vi "Destroy User Event.vi"(8 "error in (no error)":errorcluster) -> (0 "error out":errorcluster)   [LabVIEW 2017]
uses:
  Reference Action.ctl
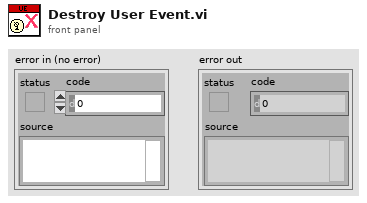
[diagram p1: front panel]
types:
  T1 = typedef "Reference Action.ctl" = enum16{"Set", "Get"}
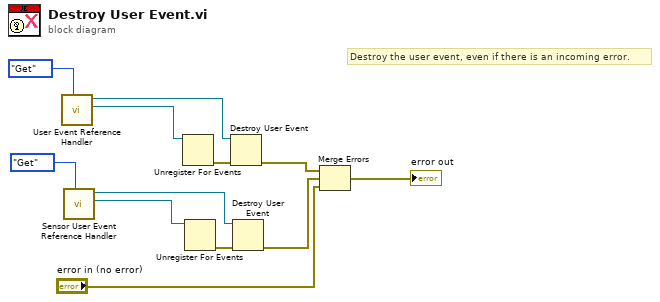
[diagram p0: block diagram]
diagram:
  # "Destroy the user event, even if there is an incoming error."
  n1 = call "User Event Reference Handler.vi"("Reference Action"=Reference_Action."Get") -> ("Event Registration Refnum Out"=w10:refnum<event-registration>, "User Event Refnum Out"=w9:refnum<user-event>)  [unwired: 8 in, 1 out]
  n2 = call "Sensor User Event Reference Handler.vi"("Reference Action"=Reference_Action."Get") -> ("Event Registration Refnum Out"=w3:refnum<event-registration>, "User Event Refnum Out"=w4:refnum<user-event>)  [unwired: 8 in, 1 out]
  n3 = Unregister For Events(event registration refnum=w10) -> (error out=w8:errorcluster)  [unwired: 1 in]
  n4 = Unregister For Events(event registration refnum=w3) -> (error out=w5:errorcluster)  [unwired: 1 in]
  n5 = Destroy User Event(user event=w9, error in=w8) -> (error out=w7:errorcluster)
  n6 = Destroy User Event(user event=w4, error in=w5) -> (error out=w2:errorcluster)
  n7 = Merge Errors(w7, w2, "error in (no error)") -> (→"error out":errorcluster)
